vi "Size.vi"(8 "error in (no error)":errorcluster, 11 "Waveform Array in":refnum<class "Waveform Array.lvclass">) -> (0 "error out":errorcluster, 2 "Size":i32, 3 "Waveform Array out":refnum<class "Waveform Array.lvclass">)   [LabVIEW 2020, in "Data.lvlib" / "Waveform Array.lvclass"]
doc: "Return the size of the generic data element."
uses:
  Waveform Array.lvclass
  Waveform Array.lvclass/Waveform Array.ctl
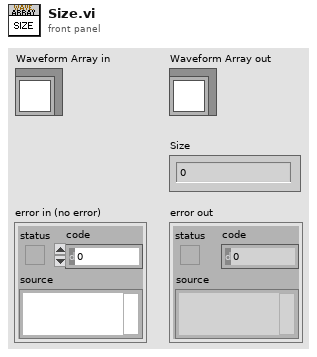
[diagram p1: front panel]
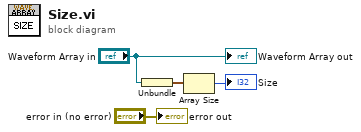
[diagram p0: block diagram]
diagram:
  n1 = Unbundle("Waveform Array in") -> (w2:waveform(dbl)[])
  n2 = Array Size(array=w2) -> (size(s)=→"Size":i32)
  "error out" <- "error in (no error)"
  "Waveform Array out" <- "Waveform Array in"
